vi "Load.vi"(0 "LV MDI.lvclass":refnum<class "LV MDI.lvclass">, 7 "Vi Path":path=path "C:/Users/namratha.balakrishna/Documents/LabVIEW Data/MDI/source code/Labview MDI/Example/Waveform.vi", 11 "error in (no error)":errorcluster) -> (4 "LV MDI.lvclass":refnum<class "LV MDI.lvclass">, 6 "Name[]":string[](array[string]), 15 "error out":errorcluster)   [LabVIEW 2016, in "LV MDI.lvclass"]
uses:
  LV MDI.lvclass
  LV MDI.lvclass/LV MDI.ctl
  Document/Document.lvclass
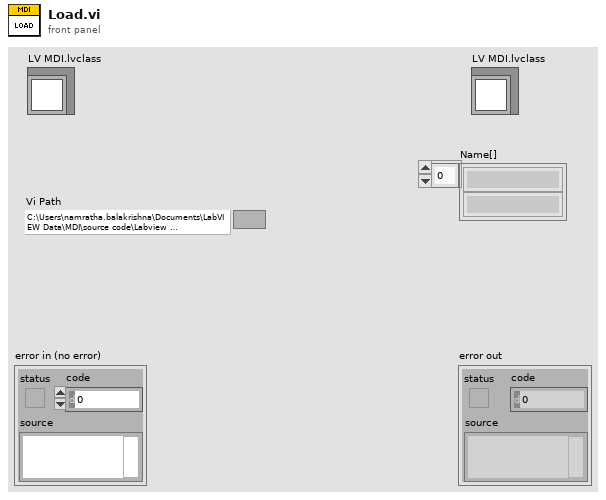
[diagram p1: front panel]
types:
  T1 = typedef "LV MDI.lvclass/Child Window Data.ctl" = cluster{"Child hWnd":u32, "UID":string, "Name":string}
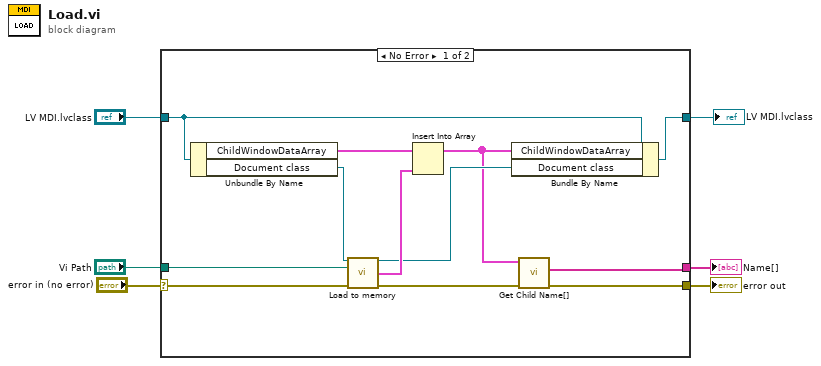
[diagram p0: block diagram]
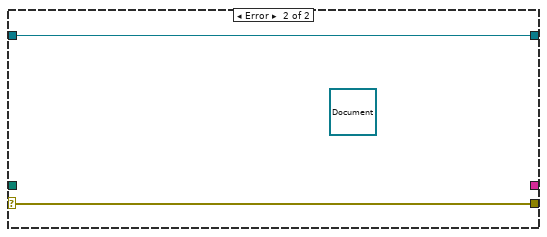
[diagram p2: hidden frame]
diagram:
  n1 = case shown="No Error" "error in (no error)" {
    selector: "error in (no error)" -> [w18 w20]
    tunnel: [w10 w20] -> w5
    tunnel: "Vi Path" -> [w7 _]
    tunnel: [w8 _] -> w3
    tunnel: [w15 w19] -> w1
    tunnel: "LV MDI.lvclass" -> [w16 w19]
    frame No Error {
      n2 = Unbundle By Name(w16) -> ("ChildWindowDataArray"=w14:T1[], "Document class"=w17:refnum<class "Document.lvclass">)
      n3 = call-dynamic "Load to memory.vi"("Document in"=w17, "Path"=w7, "error in (no error)"=w18) -> ("Document out"=w12:refnum<class "Document.lvclass">, "Child Window Data"=w13:T1, "error out"=w11:errorcluster)  [unwired: 10 in]
      n4 = Insert Into Array(array=w14, new element=w13) -> (w9:T1[])  [unwired: 1 in]
      n5 = Bundle By Name(cluster=w16, "ChildWindowDataArray"=w9, "Document class"=w12) -> (w15:refnum<class "LV MDI.lvclass">)
      n6 = call "Get Child Name[].vi"("error in (no error)"=w11, "output array"=w9) -> ("error out"=w10:errorcluster, "Array"=w8:string[])  [unwired: 8 in]
    }
    frame Error {
      (unwired) refnum<class "Document.lvclass"> refnum ("Document out")
    }
  }
  "error out" <- w5
  "Name[]" <- w3
  "LV MDI.lvclass" <- w1
